vi "Example Simple.vi"() -> ()   [LabVIEW 2014]
doc: "This examples shows off many of the basic usage patterns of the datagrid."
uses:
  System.Windows.Forms
  GridColumn/ColumnDefinition.ctl
  GridColumn/ColumnType.ctl
  DataGridView/DataGridView.lvclass
  DataGrid.lvlib
  GridColumn/GridColumn.lvclass
panel:
  out "Events":string
  in  "# of Rows":i32=15
  in  "ColumnSetup":T1[](array[typedef])=[{"name"="Text", "caption"="Text", "datatype"=enum."string", "Params"="", "AutoSizeMode"=16, "FillWeight"=15.0, "MinWidth"=40}, {"name"="Details", "caption"="Text", "datatype"=enum."string", "Params"="", "AutoSizeMode"=16, "FillWeight"=85.0, "MinWidth"=150}, {"name"="Time", "caption"="", "datatype"=enum."timestamp", "Params"="", "AutoSizeMode"=1, "FillWeight"=1.0, "MinWidth"=120}, {"name"="Selection", "caption"="", "datatype"=enum."combo", "Params"="One|Two|Three", "AutoSizeMode"=6, "FillWeight"=1.0, "MinWidth"=80}, {"name"="Function", "caption"="", "datatype"=enum."button", "Params"="", "AutoSizeMode"=6, "FillWeight"=1.0, "MinWidth"=50}, {"name"="Value", "caption"="", "datatype"=enum."numeric", "Params"="", "AutoSizeMode"=6, "FillWeight"=1.0, "MinWidth"=10}, {"name"="Active", "caption"="", "datatype"=enum."check", "Params"="", "AutoSizeMode"=6, "FillWeight"=1.0, "MinWidth"=10}, {"name"="Status", "caption"="", "datatype"=enum."image", "Params"="", "AutoSizeMode"=6, "FillWeight"=1.0, "MinWidth"=10}, {"name"="Link", "caption"="", "datatype"=enum."link", "Params"="", "AutoSizeMode"=1, "FillWeight"=100.0, "MinWidth"=50}] {"MinWidth" min=2 step=1; "AutoSizeMode" items=["None"=1, "ColumnHeader"=2, "AllCellsExceptHeader"=4, "AllCells"=6, "DisplayedCellsExceptHeader"=8, "DisplayedCells"=10, "Fill"=16]; "FillWeight" min=1 max=100}
  in  "DataGridView":refnum<k24>(container)
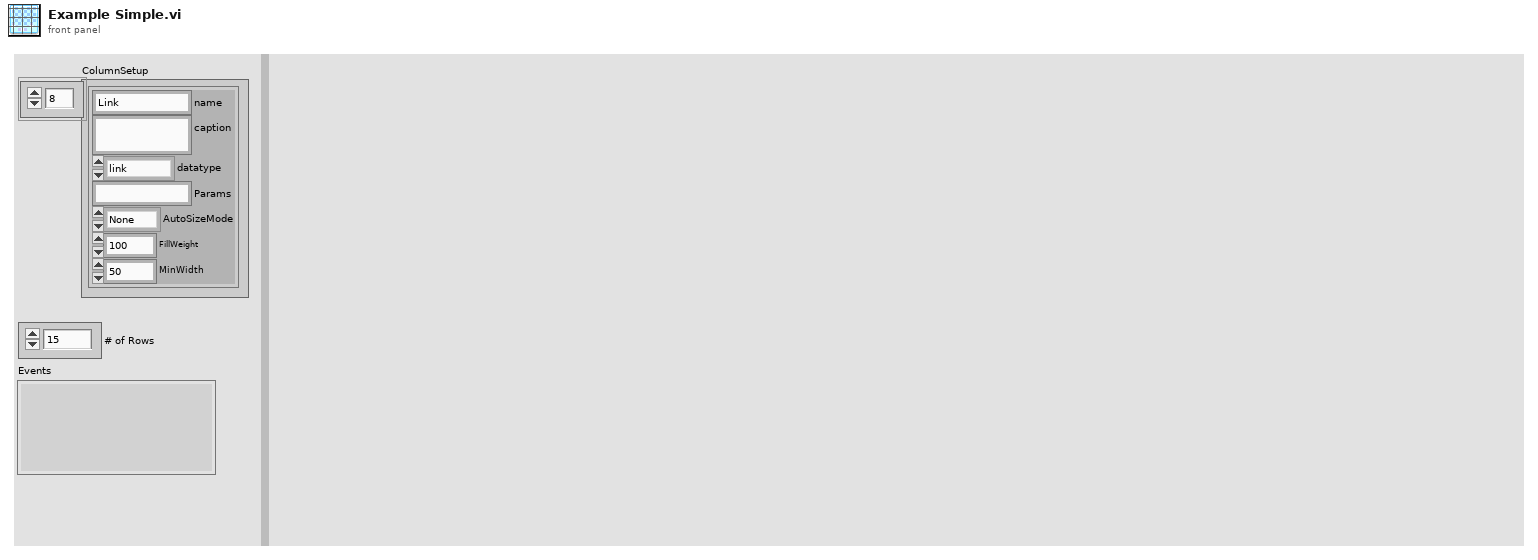
[diagram p1: front panel]
types:
  T1 = typedef "DataGrid.lvlib/GridColumn.lvclass/ColumnDefinition.ctl" = cluster{"name":string, "caption":string, "datatype":T2, "Params":string, "AutoSizeMode":i32, "FillWeight":sgl, "MinWidth":u32}
  T2 = typedef "DataGrid.lvlib/GridColumn.lvclass/ColumnType.ctl" = enum16{"string", "image", "check", "numeric", "timestamp", "button", "combo", "link"}
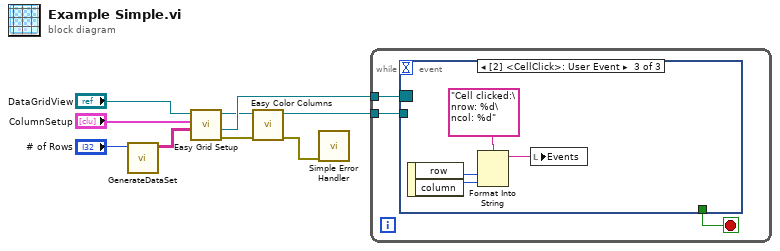
[diagram p0: block diagram]
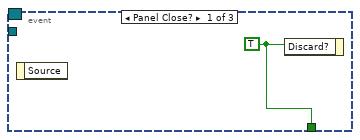
[diagram p2: hidden frame]
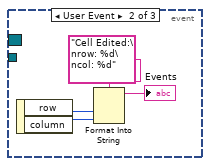
[diagram p3: hidden frame]
diagram:
  n1 = call "GenerateDataSet.vi"("Records"="# of Rows") -> ("DataGrid"=w6:string[][])  [unwired: 10 in]
  n2 = call "Easy Grid Setup.vi"("DataSource Data"=w6, "ColumnSetup"="ColumnSetup", ".net datagridview ref"="DataGridView") -> ("error out"=w4:errorcluster, "Grid RegisteredEvents"=w5:refnum<event-registration>, "DataGrid out"=w2:refnum<class "DataGridView.lvclass">)  [unwired: 5 in, 1 out]
  n3 = call "Easy Color Columns.vi"("error in (no error)"=w4, "DataGridView in"=w2) -> ("error out"=w3:errorcluster, "DataGridView out"=w1:refnum<class "DataGridView.lvclass">)  [unwired: 8 in]
  n4 = call <vilib>:"Simple Error Handler.vi"("error in (no error)"=w3) -> ()  [unwired: 4 in, 5 out]
  n5 = while {
    tunnel: w5 -> [w11]
    tunnel: w1 -> [w10]
    stop <- w12 stop-if-true
    n6 = event shown="[2] <CellClick>: User Event" {
      selector: w11 -> [_ _ _]
      dyn-events: _ -> [_ _ _]
      timeout: _ -> [_ _ _]
      tunnel: [w13 _ _] -> w12
      tunnel: w10 -> [_ _ _]
      event Panel Close? {
        w13 = TRUE ("Discard?")
        n7 = event-data() -> ()  [unwired: 1 in, 1 out]
        n8 = event-data("Discard?"=w13) -> ()  [unwired: 1 in, 1 out]
      }
      event User Event {
        n9 = event-data() -> ("row"=w15:i32, "column"=w16:i32)  [unwired: 1 in]
        n10 = Format Into String(format string="Cell Edited:\nrow: %d\ncol: %d" ("message"), w15, w16) -> (resulting string=→"Events":string)  [unwired: 2 in, 1 out]
      }
      event User Event {
        n11 = event-data() -> ("row"=w19:i32, "column"=w20:i32)  [unwired: 1 in]
        n12 = Format Into String(format string="Cell clicked:\nrow: %d\ncol: %d" ("message"), w19, w20) -> (resulting string=w18:string)  [unwired: 2 in, 1 out]
        n13 = local write "Events"(w18) -> ()
      }
    }
  }
